vi "client.vi"() -> ()   [LabVIEW 2018]
panel:
  in  "设备信息":T1
  in  "停止":bool
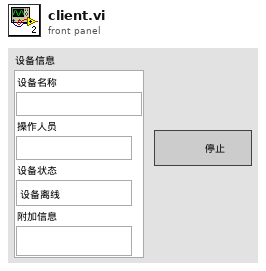
[diagram p1: front panel]
types:
  T1 = cluster{"设备名称":string, "操作人员":string, "设备状态":enum16{"设备离线", "设备正常", "设备缺料", "设备故障", "质量报警"}, "附加信息":string}
  T2 = cluster{"设备名称":bool, "操作人员":bool, "设备状态":bool, "附加信息":bool}
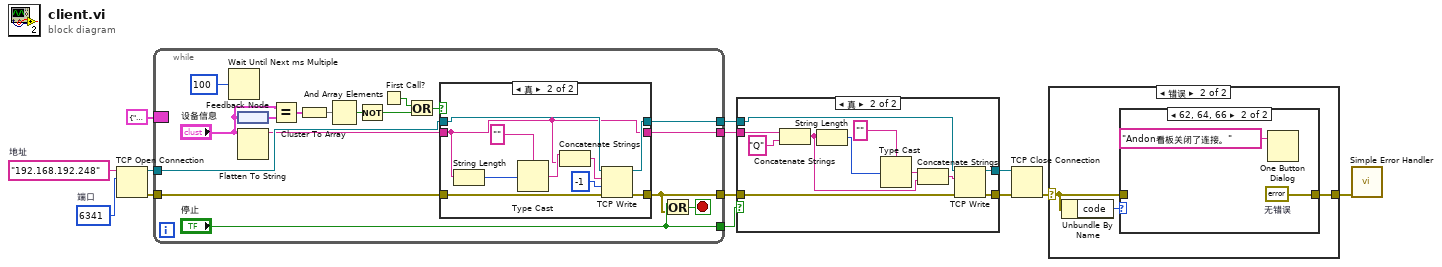
[diagram p0: block diagram]
diagram:
  w12 = u16 6341  # 端口
  w13 = "192.168.192.248"  # 地址
  n1 = TCP Open Connection(address=w13, remote port or service name=w12) -> (connection ID=w11:refnum<k5>, error out=w10:errorcluster)  [unwired: 1 in, 2 out]
  n2 = while {
    tunnel: ["停止"] -> w5
    tunnel: [w28] -> w9
    tunnel: [w25] -> w7
    tunnel: w10 -> [w29]
    tunnel: w11 -> [w30]
    tunnel: [w18] -> w2
    border: T1 {"设备名称"="", "操作人员"="", "设备状态"=enum."设备正常", "附加信息"=""} ("设备信息") -> [_]
    stop <- w27 stop-if-true
    n3 = Wait Until Next ms Multiple(millisecond multiple=u32 100 ("毫秒倍数")) -> ()  [unwired: 1 out]
    n4 = feedback-in #1("设备信息") -> ()
    n5 = feedback #1() -> (w22:T1)
    n6 = Flatten To String(anything="设备信息") -> (data string=w19:string)  [unwired: 3 in, 2 out]
    n7 = Equal?(x="设备信息", y=w22) -> (x = y?=w21:T2)
    n8 = Cluster To Array(cluster=w21) -> (array=w20:bool[])
    n9 = And Array Elements(Boolean array=w20) -> (logical AND=w17:bool)
    n10 = Not(x=w17) -> (.not. x?=w14:bool)
    n11 = First Call?() -> (First Call?: T/F=w15:bool)
    n12 = Or(x=w15, y=w14) -> (x .or. y?=w16:bool)
    n13 = case shown="真" w16 {
      tunnel: w30 -> [w33 w43]
      tunnel: w29 -> [w32 w42]
      tunnel: [w33 w41] -> w28
      tunnel: [w32 w40] -> w25
      tunnel: w19 -> [w31 w34]
      tunnel: [w31 w34] -> w18
      frame False {
      }
      frame True {
        n14 = String Length(string=w34) -> (length=w38:i32)
        n15 = Type Cast(type="", x=w38) -> (*(type *) &x=w36:string)
        n16 = Concatenate Strings(w36, w34) -> (w35:string)
        n17 = TCP Write(connection ID=w43, data in=w35, error in (no error)=w42, 9:-1) -> (connection ID out=w41:refnum<k5>, error out=w40:errorcluster)  [unwired: 1 out]
      }
    }
    n18 = Or(x="停止", y=w25) -> (x .or. y?=w27:bool)
  }
  n19 = case shown="真" w5 {
    tunnel: w9 -> [w45 w56]
    tunnel: [w45 w54] -> w8
    tunnel: w7 -> [w44 w55]
    tunnel: [w44 w53] -> w6
    tunnel: w2 -> [_ w51]
    frame False {
    }
    frame True {
      n20 = Concatenate Strings(w51, "Q") -> (w47:string)
      n21 = String Length(string=w47) -> (length=w50:i32)
      n22 = Type Cast(type="", x=w50) -> (*(type *) &x=w48:string)
      n23 = Concatenate Strings(w48, w47) -> (w46:string)
      n24 = TCP Write(connection ID=w56, data in=w46, error in (no error)=w55) -> (connection ID out=w54:refnum<k5>, error out=w53:errorcluster)  [unwired: 2 out]
    }
  }
  n25 = TCP Close Connection(connection ID=w8, error in (no error)=w6) -> (error out=w4:errorcluster)  [unwired: 2 out]
  n26 = case shown="错误" w4 {
    selector: w4 -> [w57 w59]
    tunnel: [w57 w58] -> w3
    frame No Error {
    }
    frame Error {
      n27 = Unbundle By Name(w59) -> ("code"=w60:i32)
      n28 = case shown="62, 64, 66" w60 {
        tunnel: w59 -> [w61 _]
        tunnel: [w61 w63] -> w58
        frame Default {
        }
        frame 62, 64, 66 {
          w63 = errorcluster {"status"=FALSE, "code"=0, "source"=""}  # 无错误
          n29 = One Button Dialog(message="Andon看板关闭了连接。" ("服务器关闭")) -> ()  [unwired: 1 in, 1 out]
        }
      }
    }
  }
  n30 = call <vilib>:"Simple Error Handler.vi"("error in (no error)"=w3) -> ()  [unwired: 1 in, 8 out]
